vi "CheckSchemaVersion.vi"(8 "error in (no error)":errorcluster, 10 "ValidSchemaVersions":string[](array[string])=["0.0.1"], 11 "schemaVersionIn":string) -> (0 "error out":errorcluster, 2 "CurrentSchemaVersion":string, 3 "schemaVersionOut":string)   [LabVIEW 2026, in "Lumberjack.lvlib"]
doc: "Validates a config's schema version against the accepted set.\nPasses schemaVersionIn through as schemaVersionOut when it is a member of ValidSchemaVersions; an omitted key reads as CurrentSchemaVersion so a config without the key is treated as current; an unrecognized version is rejected so the validator can refuse configs it does not understand (SDD 4.2). No I/O.\nLumberjack.lvlib, community (friend of Tests.lvlib)."
uses:
  Lumberjack.lvlib
  <vilib>/AdvancedString/1D String Array to Delimited String (string).vi
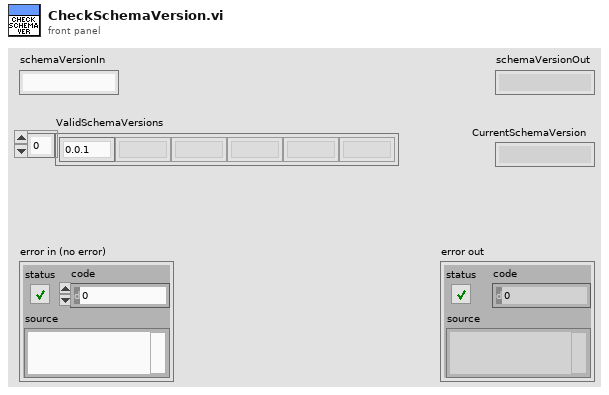
[diagram p1: front panel]
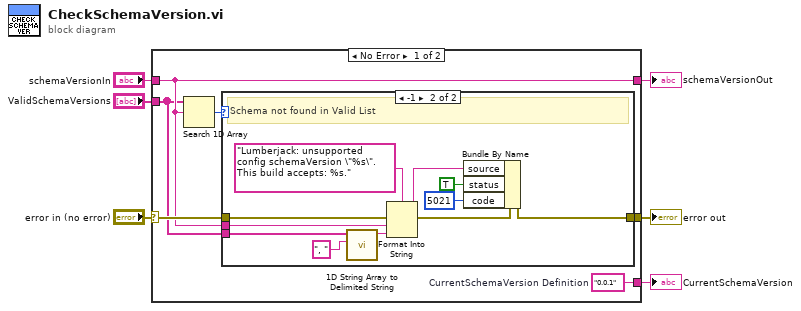
[diagram p0: block diagram]
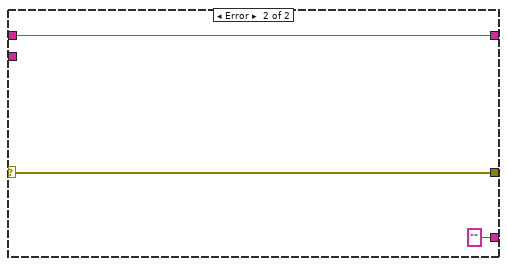
[diagram p3: hidden frame]
diagram:
  n1 = case shown="No Error" "error in (no error)" {
    selector: "error in (no error)" -> [w10 w27]
    tunnel: [w12 w27] -> w6
    tunnel: "schemaVersionIn" -> [w9 w26]
    tunnel: "ValidSchemaVersions" -> [w8 _]
    tunnel: [w9 w26] -> w2
    tunnel: [w7 "" ("schemaVersion")] -> w1
    frame No Error {
      w7 = "0.0.1"  # CurrentSchemaVersion Definition
      n2 = Search 1D Array(1D array=w8, element=w9) -> (index of element=w11:i32)  [unwired: 1 in]
      n3 = case shown="-1" w11 {
        tunnel: w10 -> [w13 w21]
        tunnel: [w13 w24] -> w12
        tunnel: w9 -> [_ w18]
        tunnel: w8 -> [_ w17]
        frame Default {
          # "Schema found in Valid List"
        }
        frame -1 {
          # "Schema not found in Valid List"
          n4 = call-poly <vilib>:"1D String Array to Delimited String.vi"("delimiter"=", ", "string array"=w17) -> ("delimited string"=w15:string)  [unwired: 9 in]
          n5 = Format Into String(format string="Lumberjack: unsupported config schemaVersion \"%s\". This build accepts: %s." ("source"), error in=w21, w18, w15) -> (resulting string=w19:string, error out=w20:errorcluster)  [unwired: 1 in]
          n6 = Bundle By Name(cluster=w20, "source"=w19, "status"=TRUE, "code"=5021) -> (w24:errorcluster)
        }
      }
    }
    frame Error {
    }
  }
  "error out" <- w6
  "schemaVersionOut" <- w2
  "CurrentSchemaVersion" <- w1
